vi "send_voltageStep-v02.vi"(0 "daq_ao":tag="Dev1/ao1", 1 "daq_ai":tag="Dev1/ai0:1", 5 "VoltageStepValuesCluster":T2, 7 "Sample Freq (Hz)":dbl min=0.0 max=40000.0, 9 "set holding (mV)":dbl, 13 "Number of Replicates":i16=1 min=1 max=10, 14 "error in":errorcluster) -> (4 "output cluster":T1, 6 "output waveform":waveform(dbl)[](graph), 8 "protocol response":waveform(dbl)[](graph) caption="jumptestMonitor", 10 "error out":errorcluster)   [LabVIEW 2019]
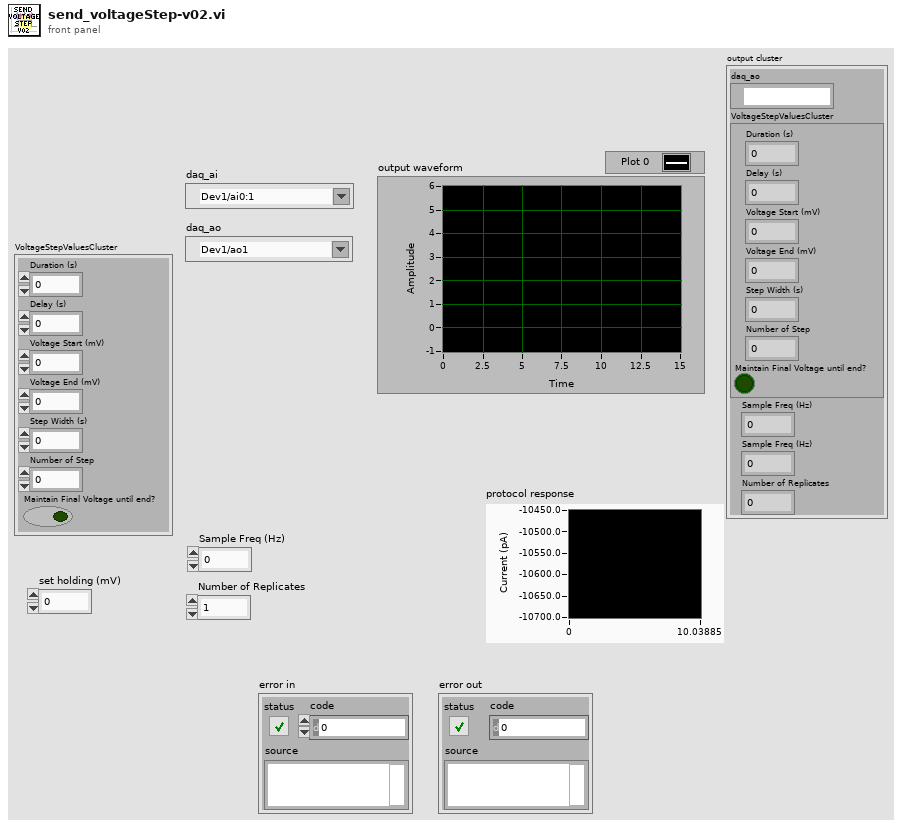
[diagram p1: front panel]
types:
  T1 = cluster{"daq_ao":tag, "VoltageStepValuesCluster":cluster{"Duration (s)":dbl, "Delay (s)":dbl, "Voltage Start (mV)":dbl, "Voltage End (mV)":dbl, "Step Width (s)":dbl, "Number of Step":dbl, "Maintain Final Voltage until end?":bool}, "Sample Freq (Hz)":dbl, "Sample Freq (Hz)":dbl, "Number of Replicates":i16}
  T2 = cluster{"Duration (s)":dbl, "Delay (s)":dbl, "Voltage Start (mV)":dbl, "Voltage End (mV)":dbl, "Step Width (s)":dbl, "Number of Step":dbl, "Maintain Final Voltage until end?":bool}
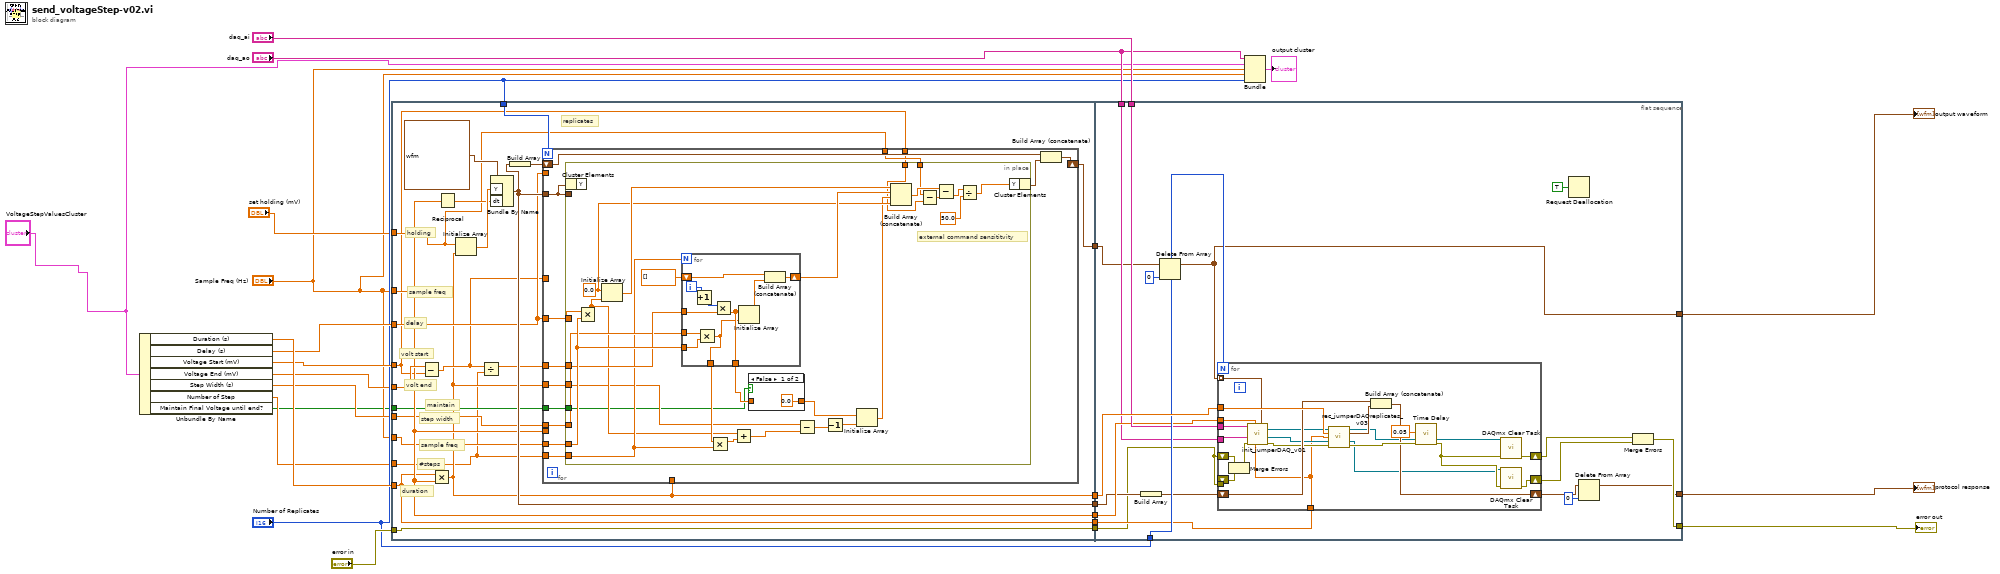
[diagram p0: block diagram]
diagram:
  n1 = Unbundle By Name("VoltageStepValuesCluster") -> ("Duration (s)"=w18:dbl, "Delay (s)"=w17:dbl, "Voltage Start (mV)"=w16:dbl, "Voltage End (mV)"=w7:dbl, "Step Width (s)"=w6:dbl, "Number of Step"=w5:dbl, "Maintain Final Voltage until end?"=w2:bool)
  n2 = flat-sequence {
    tunnel: w18 -> [w29]
    tunnel: "Sample Freq (Hz)" -> [w30]
    tunnel: [w28] -> w14
    tunnel: [w36] -> w13
    tunnel: [w39] -> w12
    tunnel: "error in" -> [w45]
    tunnel: [w45] -> w11
    tunnel: [w29] -> w10
    tunnel: w17 -> [w35]
    tunnel: w16 -> [w27]
    tunnel: [w44] -> w9
    tunnel: "Number of Replicates" -> [w43]
    tunnel: "Sample Freq (Hz)" -> [w36]
    tunnel: "set holding (mV)" -> [w31]
    tunnel: w7 -> [w38]
    tunnel: w6 -> [w34]
    tunnel: w5 -> [w25]
    tunnel: w2 -> [w26]
    tunnel: [w102] -> w24
    tunnel: w14 -> [w116]
    tunnel: "daq_ai" -> [w108]
    tunnel: "daq_ao" -> [w105]
    tunnel: w13 -> [w107]
    tunnel: [w111] -> w21
    tunnel: "Number of Replicates" -> [w115]
    tunnel: [w114] -> w19
    tunnel: w11 -> [w99]
    tunnel: w10 -> [w109]
    tunnel: w9 -> [w103]
    tunnel: w12 -> [w106]
    frame #0 {
      # "replicates"
      # "duration"
      # "#steps"
      # "sample freq"
      # "step width"
      # "maintain"
      # "volt end"
      # "volt start"
      # "delay"
      # "sample freq"
      # "holding"
      n3 = Subtract(x=w38, y=w27) -> (x-y=w33:dbl)
      n4 = Multiply(x=w29, y=w36) -> (x*y=w28:dbl)
      n5 = Reciprocal(x=w36) -> (1/x=w32:dbl)
      n6 = Initialize Array(w31, w28) -> (w40:dbl[])
      n7 = Divide(x=w33, y=w25) -> (x/y=w37:dbl)
      n8 = Bundle By Name(cluster=waveform(dbl) {"t0"=timestamp(0 s since 1904-01-01), "dt"=1.0, "Y"=[]} ("signal out"), "Y"=w40, "dt"=w32) -> (w39:waveform(dbl))
      n9 = Build Array(w39) -> (w42:waveform(dbl)[])
      n10 = for {
        N: w43 -> [_]
        tunnel: w35 -> [_]
        shift-right: [w58] -> w44
        shift-left: w42 -> [w57]
        tunnel: w39 -> [w47]
        tunnel: w37 -> [w55]
        tunnel: w36 -> [_]
        tunnel: w35 -> [w54]
        tunnel: w34 -> [w53]
        tunnel: w33 -> [_]
        tunnel: w28 -> [_]
        tunnel: w31 -> [w50]
        tunnel: w30 -> [w56]
        tunnel: w25 -> [w52]
        tunnel: w28 -> [w51]
        tunnel: w27 -> [w49]
        tunnel: w26 -> [w48]
        n11 = in-place {
          in-place-border: w47 -> [_]
          in-place-border: w56 -> [w84]
          in-place-border: w55 -> [w83]
          in-place-border: w54 -> [w79]
          in-place-border: w53 -> [w78]
          in-place-border: w52 -> [w76]
          in-place-border: w51 -> [w70]
          in-place-border: w50 -> [w65]
          in-place-border: w49 -> [w64]
          in-place-border: w48 -> [w61]
          w75 = 0.0 ("element")
          # "external command sensititvity"
          n12 = in-place-cluster #1(w47) -> ()  [unwired: 1 out]
          n13 = Multiply(x=w79, y=w84) -> (x*y=w71:dbl)
          n14 = Initialize Array(w75, w71) -> (w85:dbl[])
          n15 = for {
            N: w76 -> [_]
            tunnel: w78 -> [w96]
            tunnel: w84 -> [w95]
            tunnel: w83 -> [w94]
            shift-right: [w92] -> w82
            shift-left: dbl[] [] -> [w91]
            tunnel: [w90] -> w63
            tunnel: [w89] -> w72
            i -> [w93]
            n16 = Increment(x=w93) -> (x+1=w88:i32)
            n17 = Multiply(x=w96, y=w95) -> (x*y=w89:dbl)
            n18 = Multiply(x=w88, y=w94) -> (x*y=w90:dbl)
            n19 = Initialize Array(w90, w89) -> (w97:dbl[])
            n20 = Build Array (concatenate)(w91, w97) -> (w92:dbl[])
          }
          n21 = Multiply(x=w72, y=w76) -> (x*y=w77:dbl)
          n22 = Add(x=w71, y=w77) -> (x+y=w80:dbl)
          n23 = case shown="False" w61 {
            tunnel: w63 -> [_ w87]
            tunnel: [0.0 w87] -> w62
            frame False {
            }
            frame True {
            }
          }
          n24 = Subtract(x=w70, y=w80) -> (x-y=w69:dbl)
          n25 = Decrement(x=w69) -> (x-1=w73:dbl)
          n26 = Initialize Array(w62, w73) -> (w74:dbl[])
          n27 = Build Array (concatenate)(w85, w82, w74, w75) -> (w67:dbl[])
          n28 = Subtract(x=w65, y=w64) -> (x-y=w66:dbl)
          n29 = Subtract(x=w67, y=w66) -> (x-y=w68:dbl[])
          n30 = Divide(x=w68, y=50.0) -> (x/y=w59:dbl[])
          n31 = in-place-cluster #1("Y"=w59) -> (w46:waveform(dbl))
        }
        n32 = Build Array (concatenate)(w57, w46) -> (w58:waveform(dbl)[])
      }
    }
    frame #1 {
      n33 = Build Array(w106) -> (w113:waveform(dbl)[])
      n34 = Delete From Array(array=w103, index=0) -> (array with subset deleted=w102:waveform(dbl)[])  [unwired: 1 in, 1 out]
      n35 = for {
        N: w115 -> [_]
        tunnel: w116 -> [w137]
        shift-right: [w135] -> w112
        shift-left: w113 -> [w134]
        tunnel: w109 -> [w127]
        tunnel: w108 -> [w133]
        tunnel: w107 -> [w132]
        tunnel: w105 -> [w131]
        tunnel: w102 -> [w126] mode=indexing
        shift-right: [w121] -> w101
        shift-left: w99 -> [w119]
        shift-right: [w120] -> w100
        shift-left: _ -> [w118]
        tunnel: w99 -> [_]
        n36 = Merge Errors(w119, w118) -> (w117:errorcluster)
        n37 = call "init_jumperDAQ_v01.vi"("protocol waveform"=w126, "Duration (s)"=w127, "Sample Freq (Hz)"=w132, "AO error in"=w117, "AO physical channels"=w131, "AI Physical Channel"=w133) -> ("AO error out"=w130:errorcluster, "AO task out"=w129:refnum<k21>, "AI task out"=w128:refnum<k21>)  [unwired: 1 in, 2 out]
        n38 = call "rec_jumperDAQreplicates_v03.vi"("AI task in"=w128, "number of samples"=w137, "Duration (s)"=w127, "AO task in"=w129, "error in"=w130) -> ("AI task out"=w123:refnum<k21>, "data out (pA or mV)"=w136:waveform(dbl), "AO task out"=w122:refnum<k21>, "error out"=w138:errorcluster)  [unwired: 7 in]
        n39 = Build Array (concatenate)(w134, w136) -> (w135:waveform(dbl)[])
        n40 = call "Time Delay"("error in (no error)"=w138, "Delay Time (s)"=0.05) -> ("error out"=w124:errorcluster)  [unwired: 9 in]
        n41 = call <vilib>:"DAQmx Clear Task.vi"("task in"=w123, "error in"=w124) -> ("error out"=w121:errorcluster)  [unwired: 13 in]
        n42 = call <vilib>:"DAQmx Clear Task.vi"("task in"=w122, "error in"=w124) -> ("error out"=w120:errorcluster)  [unwired: 13 in]
      }
      n43 = Request Deallocation(TRUE ("flag")) -> ()
      n44 = Delete From Array(array=w112, index=0) -> (array with subset deleted=w111:waveform(dbl)[])  [unwired: 1 in, 1 out]
      n45 = Merge Errors(w101, w100) -> (w114:errorcluster)
    }
  }
  n46 = Bundle("daq_ao"="daq_ao", "VoltageStepValuesCluster"="VoltageStepValuesCluster", "Sample Freq (Hz)"="Sample Freq (Hz)", "Sample Freq (Hz)"="Sample Freq (Hz)", "Number of Replicates"="Number of Replicates") -> (→"output cluster":T1)  [unwired: 1 in]
  "protocol response" <- w21
  "output waveform" <- w24
  "error out" <- w19
